vi "Build.vi"(8 "error in (no error)":errorcluster, 11 "Class in":refnum<class "IB_MSI.lvclass">) -> (0 "error out":errorcluster, 1 "GeneratedFiles out":path[](array[path]), 2 "GeneratedDirectories out":path[](array[path]), 3 "Class out":refnum<class "IB_MSI.lvclass">)   [LabVIEW 2020, in "IB_MSI.lvclass"]
uses:
  <vilib>/AppBuilder/IB_Classes/MSI/IB_MSI.lvclass
  <vilib>/AppBuilder/IB_Classes/MSI/IB_MSI.lvclass/IB_MSI.ctl
  <vilib>/AppBuilder/IB_Classes/Installer/Installer.lvclass
  <resource>/Framework/Providers/Builds/Installer/CDK_sTypeDef_BuildSteps.ctl
  AppLibs/distkit/MDF/NI_MDF.lvlib
  <resource>/Framework/Providers/Builds/Installer/CDK_GLOBAL_STRINGS.vi
  <vilib>/AppBuilder/AB_Log_Error_Usage_Data_Type.ctl
  e:/builds/penguin/labview/branches/2020/dev/dist/vi.lib/AppBuilder/IB_Classes/Installer/Installer.lvclass
  e:/builds/penguin/labview/branches/2020/dev/dist/vi.lib/AppBuilder/IB_Classes/MSI/IB_MSI.lvclass
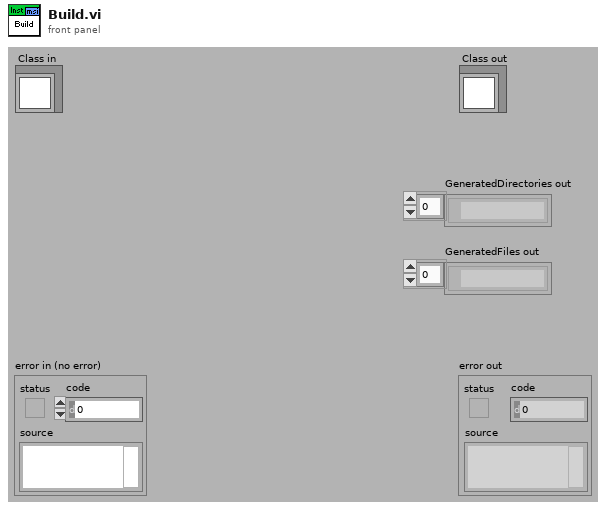
[diagram p1: front panel]
types:
  T1 = typedef "CDK_sTypeDef_BuildSteps.ctl" = enum16{"OnInitialize", "Dist_Init", "BuildDevPart", "Dist_AddParts", "Dist_Build", "OnExit"}
  T2 = typedef "AB_Log_Error_Usage_Data_Type.ctl" = enum16{"NI_APP_BUILDER_ERROR", "NI_INSTALLER_BUILDER_ERROR"}
  T3 = typedef "IB_Installer.ctl" = cluster{"Destination":refnum<class "IB_Destination.lvclass">[], "Source":refnum<class "IB_Source.lvclass">[], "buildObject":T4, "defaultDir":string, "platform":string, "author":string, "productName":string, "buildSpecName":string, "hide":bool, "requireLVDevSys":bool, "autoIncrement":bool, "includeError":bool, "readmeID":string, "buildLocation":path, "readmePath":path, "mediaSize":u16, "language":T5, "productVersion":T6, "preview":bool, "programmatic":bool, "progressBarEvents":T7, "userLog_Path":path, "shortcutAddresses":T9[], "EXE_Install Address":string, "EXE_Uninstall Address":string, "additional NIPaths":refnum<class "Dest_NI_NIPath.lvclass">[], "web service itemIDs":string[], "installerName":string}
  T4 = typedef "ItemRef.ctl" = u64
  T5 = typedef "CDK_sTypeDef_Languages.ctl" = u16
  T6 = typedef "CDK_sTypeDef_ProductVersion.ctl" = cluster{"Major":u8, "Minor":u8, "Update":u16}
  T7 = typedef "provcom_ProgressBar_Events.ctl" = cluster{"newJob":refnum<user-event>, "newItem":refnum<user-event>, "errorMsg":T8, "cancel":refnum<user-event>}
  T8 = typedef "mxLvBuildError.ctl" = refnum<user-event>
  T9 = typedef "CDK_sTypeDef_ShortcutAddress.ctl" = cluster{"file":string, "shortcut":string}
  T10 = cluster{"Event Registration Refnum":refnum<event-registration>, "newItem":refnum<user-event>, "newJob":refnum<user-event>}
  T11 = typedef "CDK_sTypeDef_DevPartInventory.ctl" = cluster{"Source":path, "FileTag":string, "RelPath":string, "Attributes":i32, "RegCOM":bool, "TargetType":T12, "shortcuts":T13[], "EXE_install":bool, "EXE_uninstall":bool, "unlock?":bool, "CmdArg_install":string, "CmdArg_uninstall":string}
  T12 = typedef "NI_MDF.lvlib/MDFBDPAddFilePathType.ctl" = i32
  T13 = typedef "CDK_sTypeDef_DevPartShortcut.ctl" = cluster{"ShortcutName":string, "SystemDirectory":string, "ProgGroup":string}
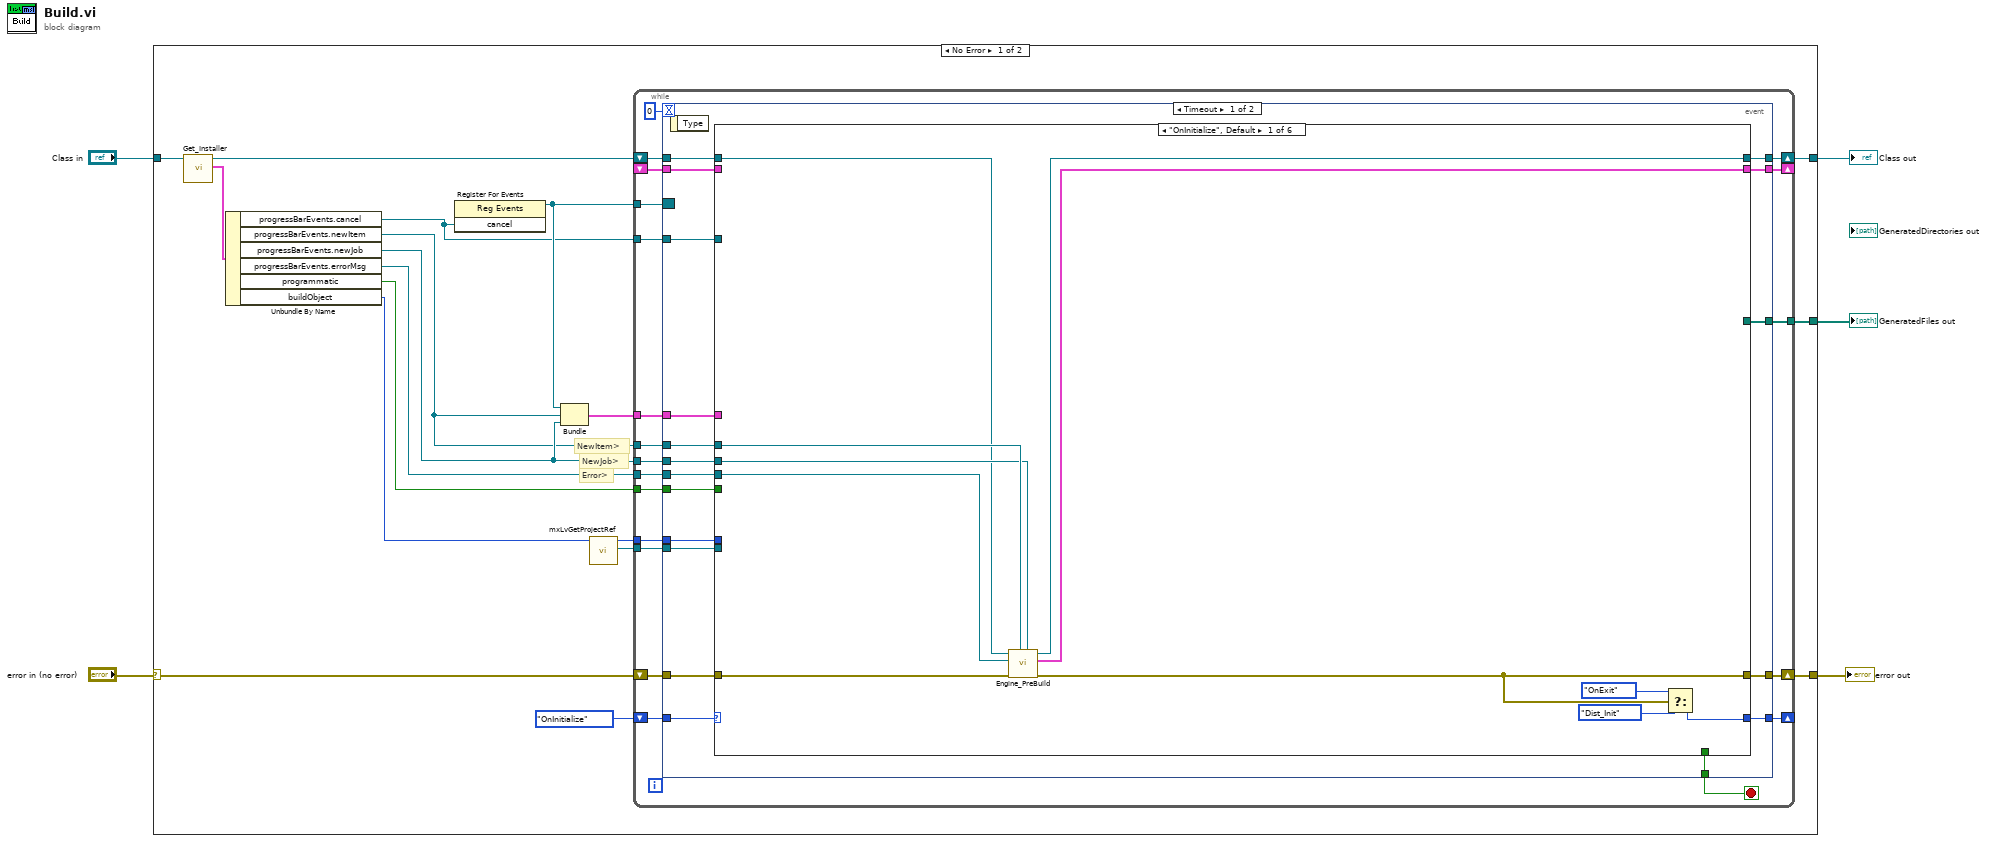
[diagram p0: block diagram]
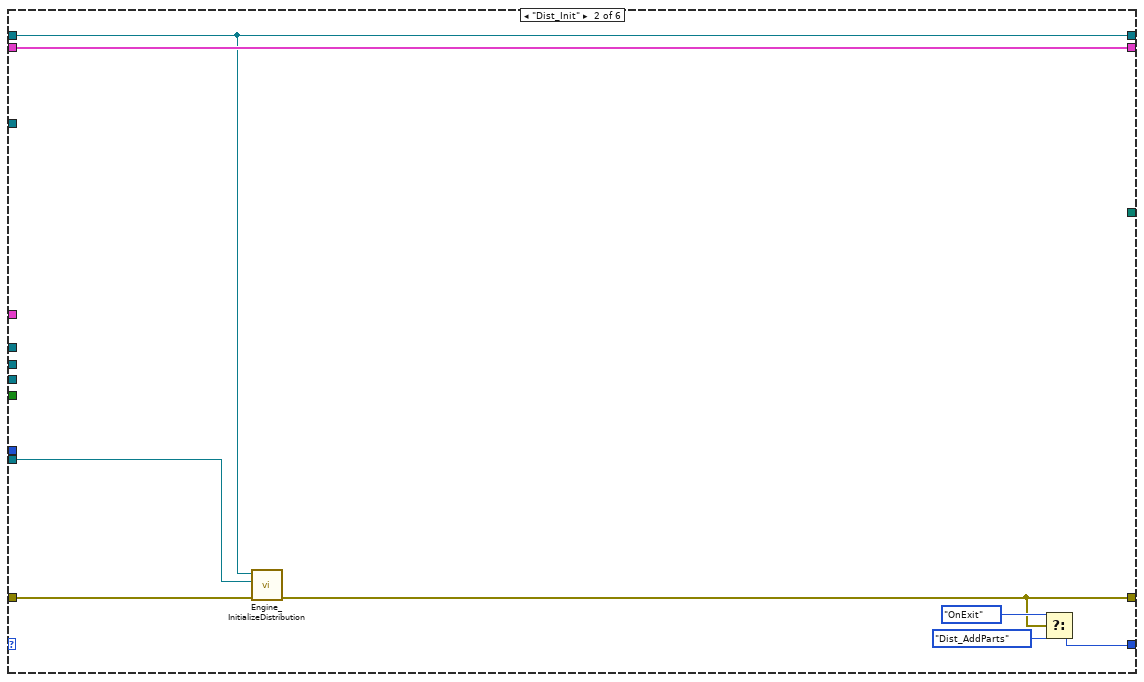
[diagram p2: hidden frame]
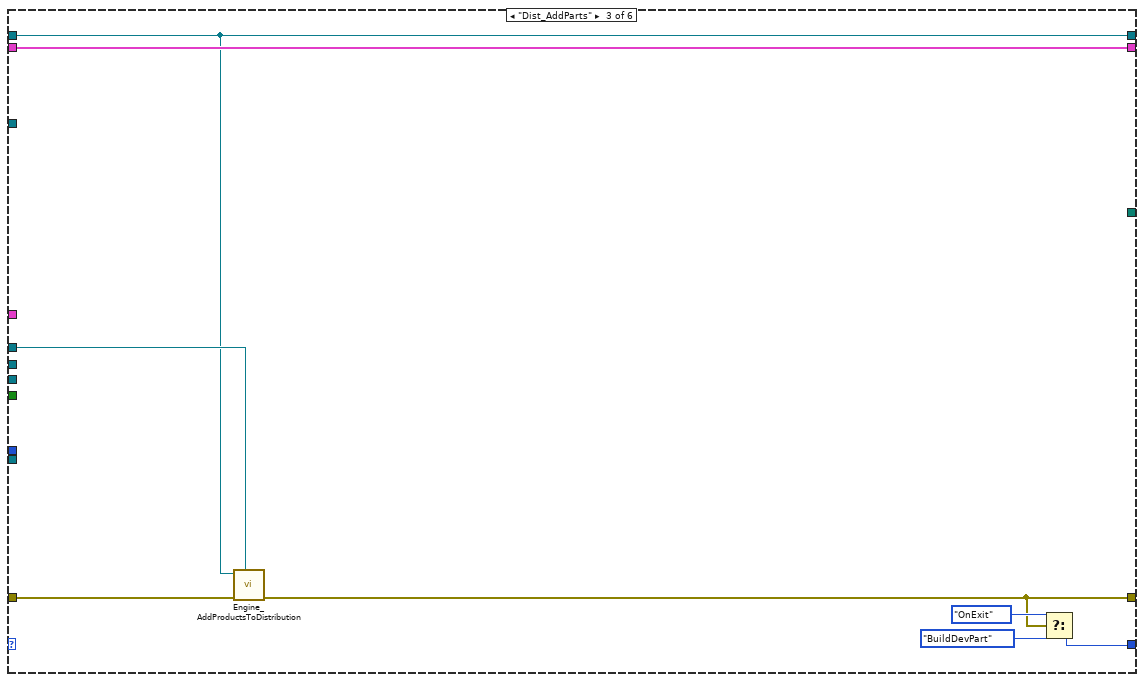
[diagram p3: hidden frame]
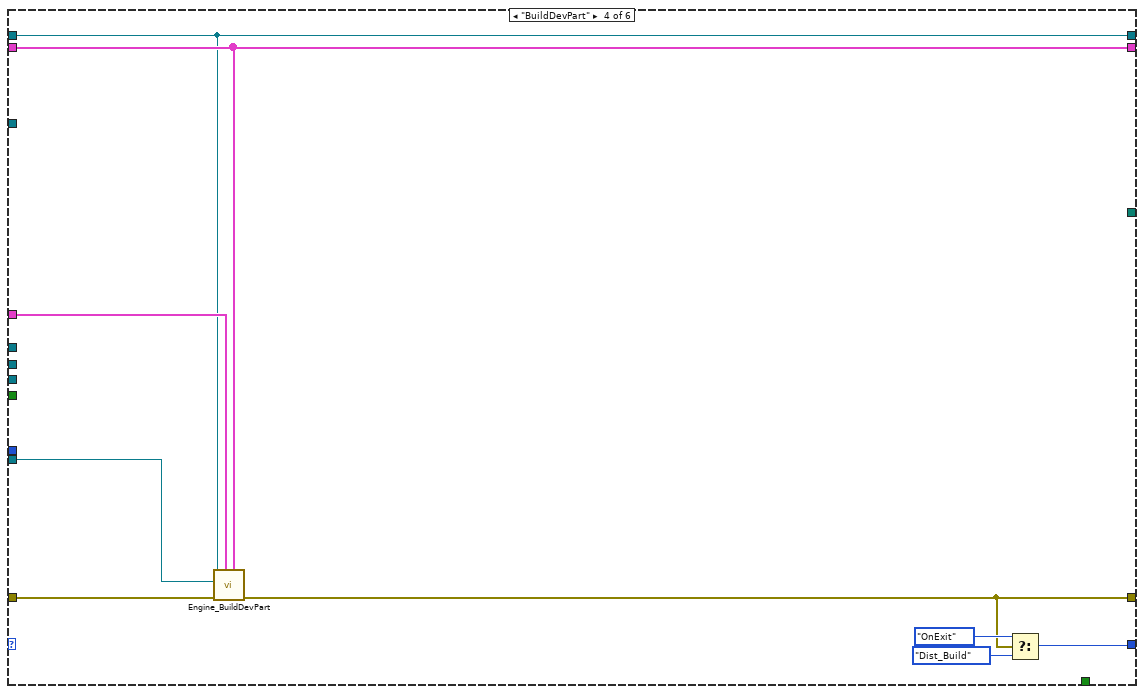
[diagram p4: hidden frame]
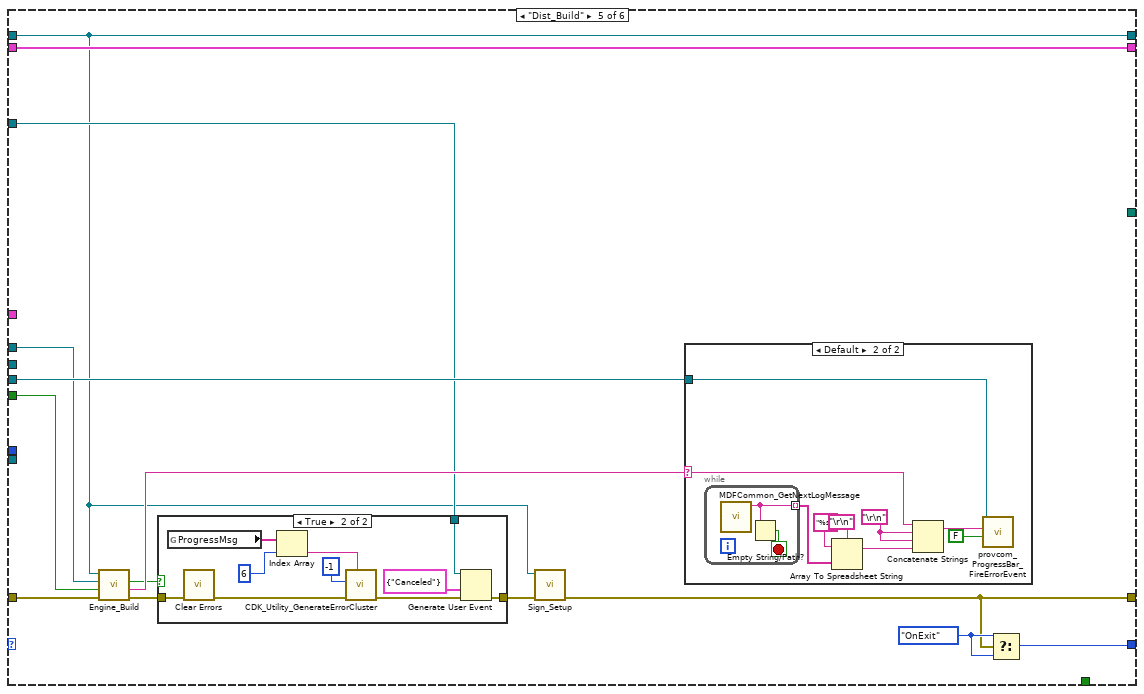
[diagram p5: hidden frame]
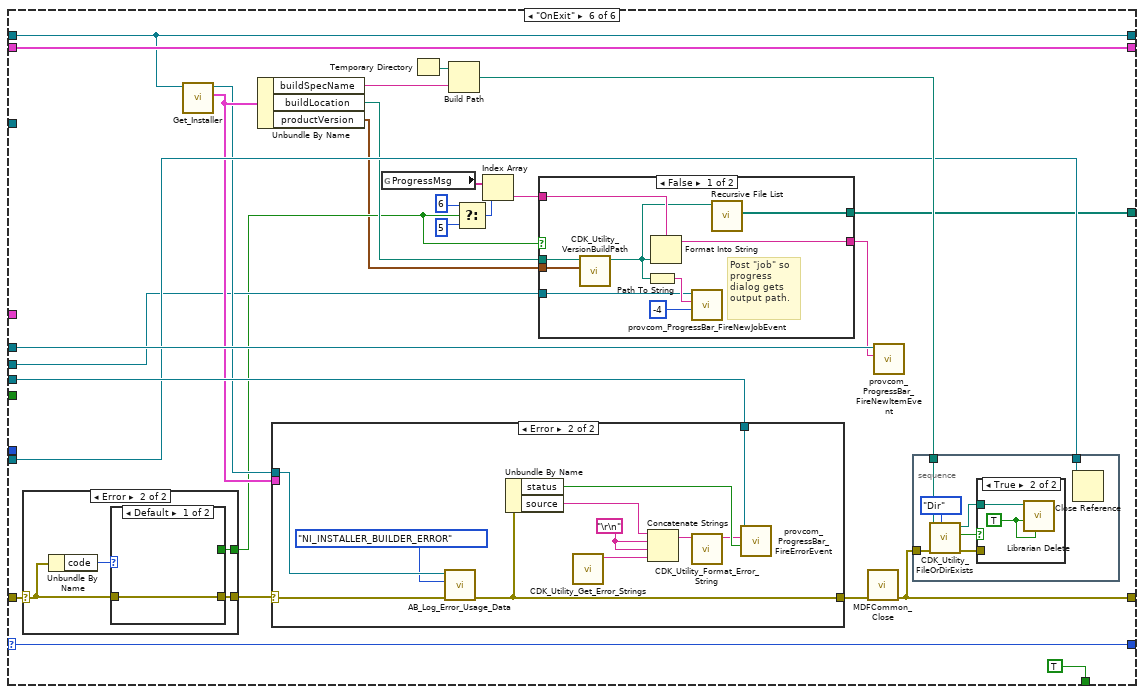
[diagram p8: hidden frame]
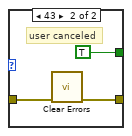
[diagram p10: hidden frame]
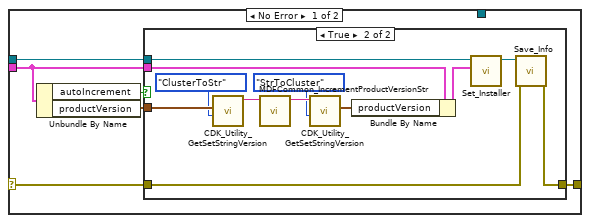
[diagram p13: hidden frame]
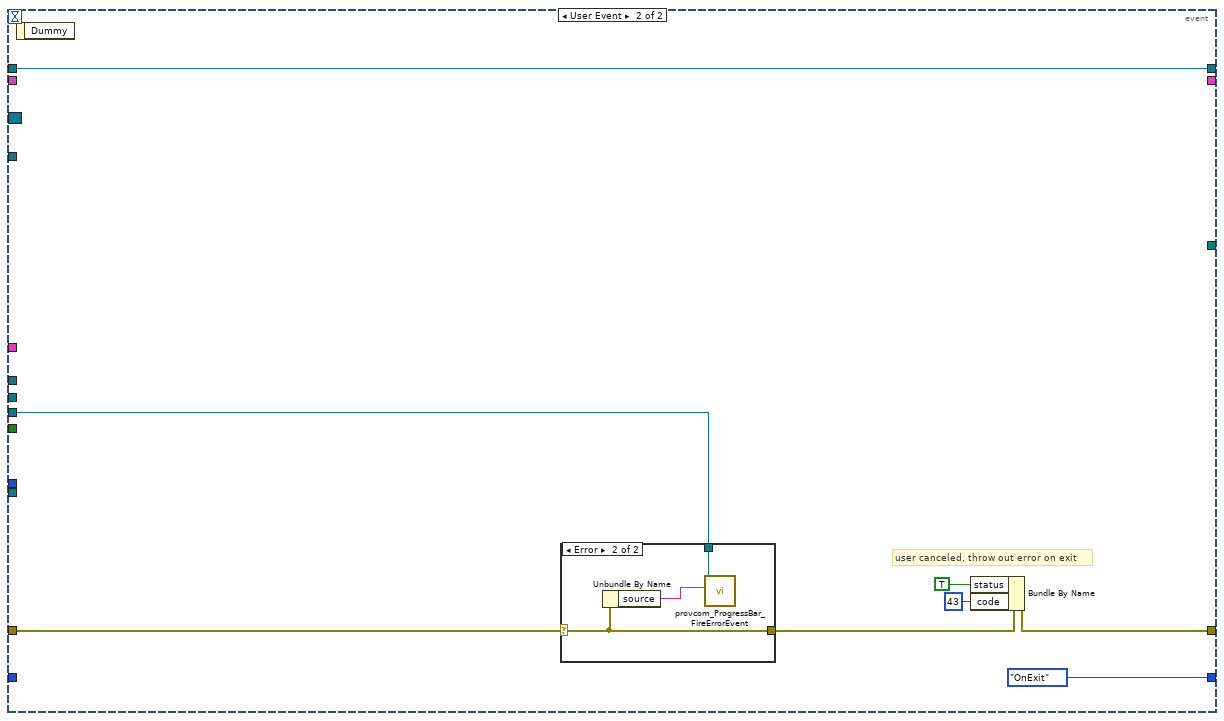
[diagram p15: hidden frame]
diagram:
  n1 = case shown="No Error" "error in (no error)" {
    selector: "error in (no error)" -> [w10 w232]
    tunnel: "Class in" -> [w14 w231]
    tunnel: [w11 w232] -> w4
    tunnel: [w7 w231] -> w2
    tunnel: [w6 _] -> w1
    frame No Error {
      # "Error>"
      # "NewJob>"
      # "NewItem>"
      n2 = call <vilib>:"Get_Installer.vi"("Installer in"=w14) -> ("data"=w13:T3, "Installer out"=w12:refnum<class "IB_MSI.lvclass">)  [unwired: 1 in, 8 out]
      n3 = Unbundle By Name(w13) -> ("progressBarEvents.cancel"=w15:refnum<user-event>, "progressBarEvents.newItem"=w16:refnum<user-event>, "progressBarEvents.newJob"=w17:refnum<user-event>, "progressBarEvents.errorMsg"=w18:T8, "programmatic"=w9:bool, "buildObject"=w8:T4)
      n4 = register-events(w15) -> (reference out=w19:refnum<event-registration>)  [unwired: 2 in, 1 out]
      n5 = Bundle("Event Registration Refnum"=w19, "newItem"=w16, "newJob"=w17) -> (w21:T10)  [unwired: 1 out]
      n6 = call <resource>:"mxLvGetProjectRef.vi"("Item"=w8) -> ("Project Refnum"=w22:refnum<vi>, "Item"=w23:T4)  [unwired: 1 in, 8 out]
      n7 = while {
        tunnel: w19 -> [w43]
        tunnel: w23 -> [w42]
        tunnel: w22 -> [w41]
        shift-right: [w38] -> w11
        shift-left: w10 -> [w39]
        tunnel: w21 -> [w37]
        shift-right: [w34] -> _
        shift-left: CDK_sTypeDef_BuildSteps."OnInitialize" ("BuildActions") -> [w36]
        shift-right: [w33] -> _
        shift-left: _ -> [w30]
        tunnel: w17 -> [w32]
        tunnel: w16 -> [w31]
        shift-right: [w29] -> w7
        shift-left: w12 -> [w28]
        tunnel: w18 -> [w27]
        tunnel: w9 -> [w26]
        tunnel: w15 -> [w25]
        tunnel: [w24] -> w6
        stop <- w35 stop-if-true
        n8 = event shown="[0] Timeout" {
          selector: w43 -> [_ _]
          dyn-events: _ -> [_ _]
          timeout: 0 -> [_ _]
          tunnel: w42 -> [w60 _]
          tunnel: w41 -> [w59 _]
          tunnel: w39 -> [w52 w226]
          tunnel: [w51 w219] -> w38
          tunnel: w37 -> [w48 _]
          tunnel: w36 -> [w61 _]
          tunnel: [w58 _] -> w35
          tunnel: [w57 CDK_sTypeDef_BuildSteps."OnExit" ("BuildActions")] -> w34
          tunnel: [w56 _] -> w33
          tunnel: w32 -> [w54 _]
          tunnel: w31 -> [w55 _]
          tunnel: w30 -> [w53 _]
          tunnel: [w50 w223] -> w29
          tunnel: w28 -> [w49 w223]
          tunnel: w27 -> [w47 w224]
          tunnel: w26 -> [w46 _]
          tunnel: w25 -> [w45 _]
          tunnel: [w44 _] -> w24
          event Timeout {
            n9 = event-data() -> ()  [unwired: 2 out]
            n10 = case shown="\"OnInitialize\", Default" w61 {
              selector: w61 -> [_ _ _ _ _ w159]
              tunnel: w60 -> [_ _ _ _ _ _]
              tunnel: w59 -> [_ w74 _ w92 _ w151]
              tunnel: [_ _ _ _ _ TRUE] -> w58
              tunnel: [w65 w78 w86 w95 w110 w159] -> w57
              tunnel: [w70 w77 w84 w96 w111 w158] -> w56
              tunnel: w55 -> [w72 _ w82 _ w101 w156]
              tunnel: w54 -> [w71 _ _ _ _ w139]
              tunnel: w53 -> [_ w77 w84 w96 w111 w158]
              tunnel: w52 -> [w69 w76 w83 w89 w109 w138]
              tunnel: [w64 w75 w85 w91 w98 w149] -> w51
              tunnel: [w68 w73 w81 w90 w99 w143] -> w50
              tunnel: w49 -> [w63 w73 w81 w90 w99 w143]
              tunnel: w48 -> [_ _ _ w97 _ _]
              tunnel: w47 -> [w62 _ _ _ w105 w155]
              tunnel: w46 -> [_ _ _ _ w107 _]
              tunnel: w45 -> [_ _ _ _ w104 _]
              tunnel: [_ _ _ _ _ w134] -> w44
              frame "OnInitialize", Default {
                n11 = call <vilib>:"Engine_PreBuild.vi"("New Job"=w71, "NewItem"=w72, "ErrIn"=w69, "errorMsg"=w62, "MSI in"=w63) -> ("ErrOut"=w64:errorcluster, "InstallerFiles"=w70:T11[], "MSI out"=w68:refnum<class "IB_MSI.lvclass">)  [unwired: 4 out]
                n12 = Select(t=CDK_sTypeDef_BuildSteps."OnExit", s=w64, f=CDK_sTypeDef_BuildSteps."Dist_Init" ("BuildActions")) -> (s? t:f=w65:T1)
              }
              frame "Dist_Init" {
                n13 = call <vilib>:"Engine_InitializeDistribution.vi"("ErrIn"=w76, "Project"=w74, "IB_MSI.lvclass"=w73) -> ("ErrOut"=w75:errorcluster)  [unwired: 8 out]
                n14 = Select(t=CDK_sTypeDef_BuildSteps."OnExit", s=w75, f=CDK_sTypeDef_BuildSteps."Dist_AddParts" ("BuildActions")) -> (s? t:f=w78:T1)
              }
              frame "Dist_AddParts" {
                n15 = call <vilib>:"Engine_AddProductsToDistribution.vi"("NewItem"=w82, "ErrIn"=w83, "IB_MSI.lvclass"=w81) -> ("ErrOut"=w85:errorcluster)  [unwired: 8 out]
                n16 = Select(t=CDK_sTypeDef_BuildSteps."OnExit", s=w85, f=CDK_sTypeDef_BuildSteps."BuildDevPart" ("BuildActions")) -> (s? t:f=w86:T1)
              }
              frame "BuildDevPart" {
                n17 = call <vilib>:"Engine_BuildDevPart.vi"("FileInventory"=w96, "EventStruct"=w97, "ErrIn"=w89, "Project"=w92, "IB_MSI.lvclass"=w90) -> ("ErrOut"=w91:errorcluster)  [unwired: 6 out]
                n18 = Select(t=CDK_sTypeDef_BuildSteps."OnExit", s=w91, f=CDK_sTypeDef_BuildSteps."Dist_Build") -> (s? t:f=w95:T1)
              }
              frame "Dist_Build" {
                w108 = CDK_sTypeDef_BuildSteps."OnExit" ("t")
                n19 = call <vilib>:"Engine_Build.vi"("ErrIn"=w109, "Programmatic?"=w107, "New item"=w101, "IB_MSI.lvclass"=w99) -> ("ErrOut"=w102:errorcluster, "warning"=w106:string, "Canceled?"=w103:bool)  [unwired: 5 out]
                n20 = case shown="True" w103 {
                  tunnel: w104 -> [_ w122]
                  tunnel: w102 -> [w112 w120]
                  tunnel: [w112 w119] -> w100
                  frame False {
                  }
                  frame True {
                    n21 = global read "CDK_GLOBAL_STRINGS.vi" "ProgressMsg"() -> (w118:string[])
                    n22 = call <vilib>:"Clear Errors.vi"("error in (no error)"=w120) -> ("error out"=w114:errorcluster)  [unwired: 1 in, 5 out]
                    n23 = Index Array(array=w118, index=6) -> (element=w115:string)
                    n24 = call <resource>:"CDK_Utility_GenerateErrorCluster.vi"("Additional Info"=w115, "ErrIn"=w114, "code"=-1) -> ("ErrOut"=w113:errorcluster)  [unwired: 1 in, 7 out]
                    n25 = Generate User Event(user event=w122, event data cluster=cluster{"Dummy":string} {"Dummy"="Canceled"} ("event data"), error in=w113) -> (error out=w119:errorcluster)  [unwired: 1 in, 1 out]
                  }
                }
                n26 = call <vilib>:"Sign_Setup.vi"("error in (no error)"=w100, "IB_MSI in"=w99) -> ("error out"=w98:errorcluster)  [unwired: 9 out]
                n27 = case shown="Default" w106 {
                  selector: w106 -> [_ w123]
                  tunnel: w105 -> [_ w124]
                  frame "" {
                  }
                  frame Default {
                    w125 = "\r\n"
                    n28 = while {
                      tunnel: [w133] -> w130 mode=indexing
                      stop <- w132 stop-if-true
                      n29 = call "MDFCommon_GetNextLogMessage.vi"() -> ("log"=w133:string)  [unwired: 1 in, 10 out]
                      n30 = Empty String/Path?(string/path=w133) -> (empty?=w132:bool)
                    }
                    n31 = Array To Spreadsheet String(delimiter (Tab)="\r\n", array=w130, 3:"%s" ("format string")) -> (spreadsheet string=w126:string)
                    n32 = Concatenate Strings(w123, w125, w125, w126) -> (w127:string)
                    n33 = call <resource>:"provcom_ProgressBar_FireErrorEvent.vi"("Error?"=FALSE, "ErrorText"=w127, "Error event"=w124) -> ()  [unwired: 1 in, 8 out]
                  }
                }
                n34 = Select(t=w108, s=w98, f=w108) -> (s? t:f=w110:T1)
              }
              frame "OnExit" {
                n35 = case shown="Error" w138 {
                  selector: w138 -> [w161 w164]
                  tunnel: [w161 w163] -> w137
                  tunnel: [_ w162] -> w136
                  frame No Error {
                  }
                  frame Error {
                    n36 = Unbundle By Name(w164) -> ("code"=w165:i32)
                    n37 = case shown="Default" w165 {
                      tunnel: w164 -> [w166 w169]
                      tunnel: [w166 w168] -> w163
                      tunnel: [_ TRUE] -> w162
                      frame Default {
                      }
                      frame 43 {
                        # "user canceled"
                        n38 = call <vilib>:"Clear Errors.vi"("error in (no error)"=w169) -> ("error out"=w168:errorcluster)  [unwired: 5 in, 1 out]
                      }
                    }
                  }
                }
                n39 = call <vilib>:"Get_Installer.vi"("Installer in"=w143) -> ("data"=w141:T3, "Installer out"=w140:refnum<class "IB_MSI.lvclass">)  [unwired: 1 in, 8 out]
                n40 = Unbundle By Name(w141) -> ("buildSpecName"=w153:string, "buildLocation"=w142:path, "productVersion"=w135:T6)
                n41 = case shown="Error" w137 {
                  selector: w137 -> [w191 w211]
                  tunnel: w155 -> [_ w218]
                  tunnel: [w194 w210] -> w150
                  tunnel: w141 -> [w190 _]
                  tunnel: w140 -> [w189 w212]
                  frame No Error {
                    n42 = Unbundle By Name(w190) -> ("autoIncrement"=w193:bool, "productVersion"=w192:T6)
                    n43 = case shown="True" w193 {
                      tunnel: w191 -> [w195 w197]
                      tunnel: [w195 w196] -> w194
                      tunnel: w192 -> [_ w207]
                      tunnel: w190 -> [_ w202]
                      tunnel: w189 -> [_ w200]
                      frame False {
                      }
                      frame True {
                        n44 = call <resource>:"CDK_Utility_GetSetStringVersion.vi"("Action"=enum16{"ClusterToStr", "StrToCluster"}."ClusterToStr", "ProductVersionIn"=w207) -> ("VersionStringOut"=w205:string)  [unwired: 2 in, 7 out]
                        n45 = call "MDFCommon_IncrementProductVersionStr.vi"("product version (1.0.0)"=w205) -> ("incremented product version"=w204:string)  [unwired: 1 in, 9 out]
                        n46 = call <resource>:"CDK_Utility_GetSetStringVersion.vi"("Action"=enum16{"ClusterToStr", "StrToCluster"}."StrToCluster", "VersionStringIn"=w204) -> ("ProductVersionOut"=w201:T6)  [unwired: 2 in, 7 out]
                        n47 = Bundle By Name(cluster=w202, "productVersion"=w201) -> (w198:T3)
                        n48 = call <vilib>:"Set_Installer.vi"("data"=w198, "Installer in"=w200) -> ("Installer out"=w199:refnum<class "IB_MSI.lvclass">)  [unwired: 1 in, 8 out]
                        n49 = call-dynamic "Save_Info.vi"("error in (no error)"=w197, "Class in"=w199) -> ("error out"=w196:errorcluster)  [unwired: 9 out]
                      }
                    }
                  }
                  frame Error {
                    w215 = "\r\n"
                    n50 = call <vilib>:"AB_Log_Error_Usage_Data.vi"("Error In"=w211, "CEIP Key (NI_APP_BUILDER_ERROR)"=AB_Log_Error_Usage_Data_Type."NI_INSTALLER_BUILDER_ERROR", "Build class"=w212) -> ("Error Out"=w210:errorcluster)  [unwired: 8 in]
                    n51 = Unbundle By Name(w210) -> ("status"=w217:bool, "source"=w216:string)
                    n52 = call <resource>:"CDK_Utility_Get_Error_Strings.vi"() -> ("error string out"=w208:string)  [unwired: 11 in]
                    n53 = Concatenate Strings(w216, w215, w215, w208) -> (w214:string)
                    n54 = call <resource>:"CDK_Utility_Format_Error_String.vi"("error string in"=w214) -> ("error string out"=w213:string)  [unwired: 10 in]
                    n55 = call <resource>:"provcom_ProgressBar_FireErrorEvent.vi"("Error?"=w217, "ErrorText"=w213, "Error event"=w218) -> ()  [unwired: 1 in, 8 out]
                  }
                }
                n56 = global read "CDK_GLOBAL_STRINGS.vi" "ProgressMsg"() -> (w157:string[])
                n57 = Temporary Directory() -> (w154:path)
                n58 = Build Path(base path=w154, name or relative path=w153) -> (appended path=w152:path)
                n59 = Select(t=6 ("index"), s=w136, f=5 ("index")) -> (s? t:f=w144:i32)
                n60 = Index Array(array=w157, index=w144) -> (element=w148:string)
                n61 = case shown="False" w136 {
                  tunnel: w148 -> [w178 w179]
                  tunnel: w142 -> [w173 _]
                  tunnel: [w177 w179] -> w147
                  tunnel: w139 -> [w174 _]
                  tunnel: w135 -> [w172 _]
                  tunnel: [w170 _] -> w134
                  frame False {
                    # "Post \"job\" so progress dialog gets output path."
                    n62 = call <resource>:"CDK_Utility_VersionBuildPath.vi"("ProductVersionIn"=w172, "build path in"=w173) -> ("build path out"=w171:path)  [unwired: 7 in, 2 out]
                    n63 = Path To String(path=w171) -> (string=w175:string)
                    n64 = Format Into String(format string=w178, w171) -> (resulting string=w177:string)  [unwired: 2 in, 1 out]
                    n65 = call <resource>:"provcom_ProgressBar_FireNewJobEvent.vi"("#ofItems"=-4, "Label"=w175, "New Job"=w174) -> ()  [unwired: 8 in, 1 out]
                    n66 = call <vilib>:"Recursive File List.vi"("Folder Path"=w171) -> ("All Files in Dir"=w170:path[])  [unwired: 6 in, 4 out]
                  }
                  frame True {
                  }
                }
                n67 = call "MDFCommon_Close.vi"("error in (no error)"=w150) -> ("error out"=w149:errorcluster)  [unwired: 10 out]
                n68 = call <resource>:"provcom_ProgressBar_FireNewItemEvent.vi"("Label"=w147, "NewItem"=w156) -> ()  [unwired: 1 in, 9 out]
                n69 = stacked-sequence {
                  tunnel: w149 -> [w186]
                  tunnel: w152 -> [w181]
                  tunnel: w151 -> [w180]
                  frame #0 {
                    n70 = call <resource>:"CDK_Utility_FileOrDirExists.vi"("Type (File)"=enum16{"File", "Dir"}."Dir", "ErrIn"=w186, "Path"=w181) -> ("ErrOut"=w183:errorcluster, "Exists?"=w184:bool, "dupPath"=w182:path)  [unwired: 6 out]
                    n71 = case shown="True" w184 {
                      tunnel: w183 -> [_ _]
                      tunnel: w182 -> [_ w187]
                      frame False {
                      }
                      frame True {
                        w188 = TRUE ("recursive? (F)")
                        n72 = call <vilib>:"Librarian Delete.vi"("keep deleting on error? (F)"=w188, "recursive? (F)"=w188, "path"=w187) -> ()  [unwired: 2 in, 7 out]
                      }
                    }
                    n73 = Close Reference(reference=w180) -> ()  [unwired: 1 in, 1 out]
                  }
                }
              }
            }
          }
          event User Event {
            # "user canceled, throw out error on exit"
            n74 = event-data() -> ()  [unwired: 2 out]
            n75 = case shown="Error" w226 {
              selector: w226 -> [w227 w229]
              tunnel: [w227 w229] -> w220
              tunnel: w224 -> [_ w228]
              frame No Error {
              }
              frame Error {
                n76 = Unbundle By Name(w229) -> ("source"=w230:string)
                n77 = call <resource>:"provcom_ProgressBar_FireErrorEvent.vi"("ErrorText"=w230, "Error event"=w228) -> ()  [unwired: 2 in, 8 out]
              }
            }
            n78 = Bundle By Name(cluster=w220, "status"=TRUE, "code"=43) -> (w219:errorcluster)
          }
        }
      }
    }
    frame Error {
    }
  }
  "error out" <- w4
  "Class out" <- w2
  "GeneratedFiles out" <- w1
